vi "Dir Watch.vi"(8 "error in (no error)":errorcluster, 11 "System Data":T1={"System"={"Active"=FALSE, "Exit"=FALSE, "Command wait"="", "Status_Time"=0, "Time_GPS"=0}, "Stepper Motor"={"Connection Reference"="", "Valid Connection"=FALSE, "Speed"=15}, "Camera Data"={"Image path"=path "", "Filenames"=[], "Filenames queue"=[]}, "Core"={"Close Panel on Exit?"=FALSE, "Current VI Reference"=refnum}} {"Stepper Motor"."Speed" scale=0.0..30.0}) -> (0 "error out":errorcluster, 2 "Event Refnum":refnum<event-registration>, 3 "System Data out":T1={"System"={"Active"=FALSE, "Exit"=FALSE, "Command wait"="", "Status_Time"=0, "Time_GPS"=0}, "Stepper Motor"={"Connection Reference"="", "Valid Connection"=FALSE, "Speed"=15}, "Camera Data"={"Image path"=path "", "Filenames"=[], "Filenames queue"=[]}, "Core"={"Close Panel on Exit?"=FALSE, "Current VI Reference"=refnum}} {"Stepper Motor"."Speed" scale=0.0..30.0})   [LabVIEW 2019]
uses:
  System Data.ctl
  Stepper Data.ctl
  Camera Data.ctl
panel:
  out "user event out":refnum<user-event>
  in  "Files":i32(listbox) caption="Files (Only files are shown, not folders)"
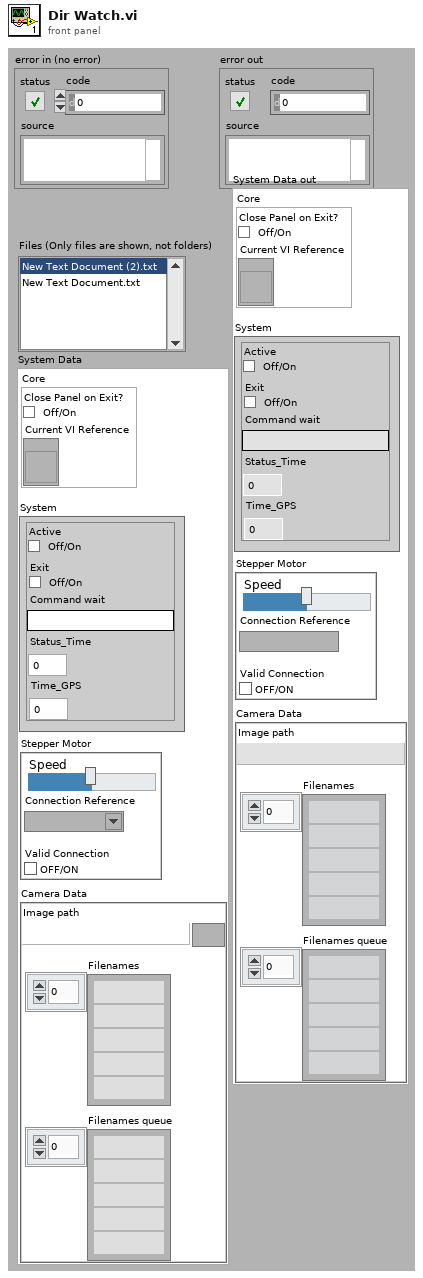
[diagram p1: front panel]
types:
  T1 = typedef "System Data.ctl" = cluster{"System":cluster{"Active":bool, "Exit":bool, "Command wait":string, "Status_Time":i32, "Time_GPS":i32}, "Stepper Motor":T2, "Camera Data":T3, "Core":cluster{"Close Panel on Exit?":bool, "Current VI Reference":refnum<vi>}}
  T2 = typedef "Stepper Data.ctl" = cluster{"Connection Reference":refnum<visa-resource-name>, "Valid Connection":bool, "Speed":i32}
  T3 = typedef "Camera Data.ctl" = cluster{"Image path":path, "Filenames":string[], "Filenames queue":string[]}
  T4 = cluster{"Dir Event":refnum<user-event>, "Image path":path}
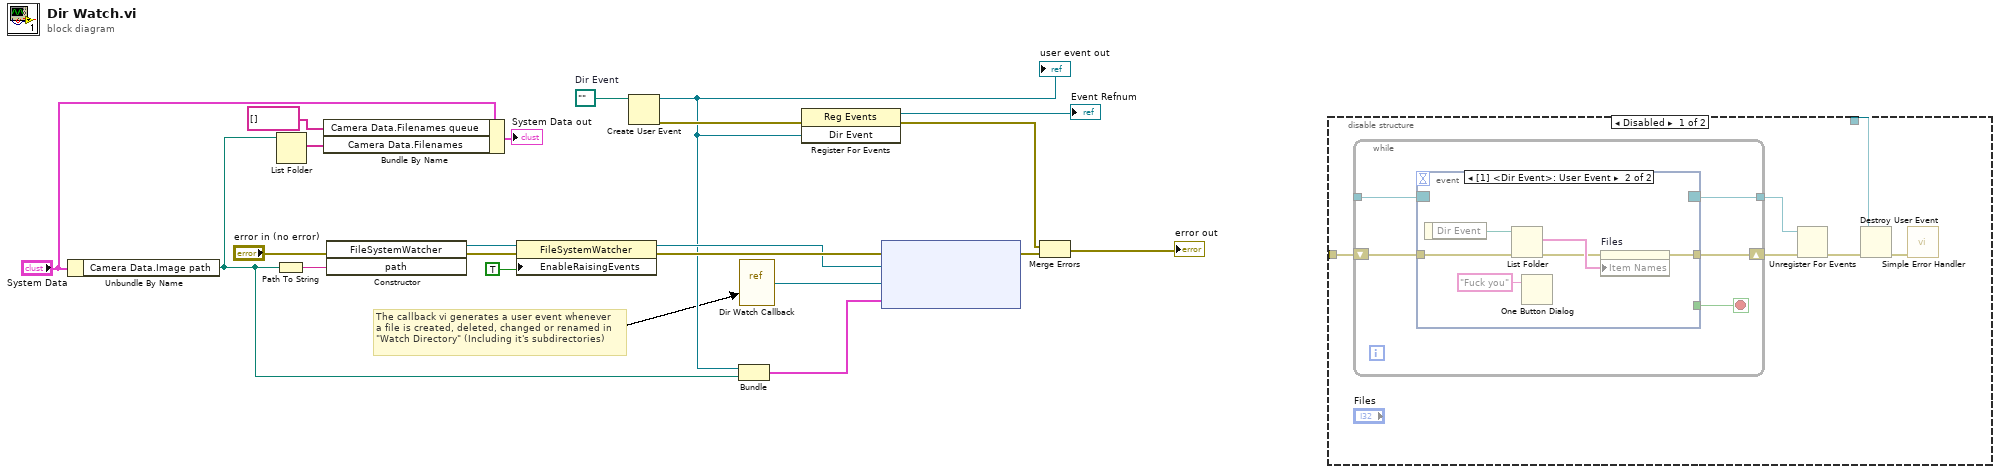
[diagram p0: block diagram]
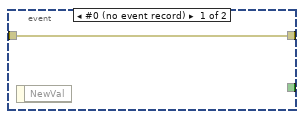
[diagram p2: hidden frame]
diagram:
  w9 = path ""  # Dir Event
  # "The callback vi generates a user event whenever\na file is created, deleted, changed or renamed in\n\"Watch Directory\" (Including it's subdirectories)"
  n1 = Unbundle By Name("System Data") -> ("Camera Data.Image path"=w5:path)
  n2 = Path To String(path=w5) -> (string=w17:string)
  n3 = List Folder(path=w5) -> (filenames=w3:string[])  [unwired: 3 in, 3 out]
  n4 = Bundle By Name(cluster="System Data", "Camera Data.Filenames queue"=string[] [], "Camera Data.Filenames"=w3) -> (→"System Data out":T1)
  n5 = constructor class="FileSystemWatcher"(error in="error in (no error)", "path"=w17) -> (reference out=w20:refnum<k24>, error out=w18:errorcluster)  [unwired: 2 in, 2 out]
  n6 = property class="FileSystemWatcher"(reference=w20, error in=w18, "EnableRaisingEvents"=TRUE) -> (reference out=w12:refnum<k24>, error out=w21:errorcluster)
  n7 = Create User Event(user event datatype=w9) -> (user event=w7:refnum<user-event>, error out=w16:errorcluster)  [unwired: 1 in]
  "user event out" <- w7
  n8 = Bundle("Dir Event"=w7, "Image path"=w5) -> (w11:T4)  [unwired: 1 in]
  n9 = vi-ref "Dir Watch Callback.vi"() -> ("vi reference"=w10:refnum<vi>)
  n10 = register-events(error in=w16, w7) -> (reference out=→"Event Refnum":refnum<event-registration>, error out=w14:errorcluster)  [unwired: 1 in]
  n11 = node(w21, w12, w10, w11) -> (w15:errorcluster)  [unwired: 1 in, 1 out]
  n12 = Merge Errors(w14, w15) -> (→"error out":errorcluster)
  n13 = disable-structure shown="Disabled" {
    disable-tunnel: _ -> [w23 _]
    disable-tunnel: _ -> [w22 _]
    frame Disabled {
      n14 = while {
        tunnel: _ -> [w31]
        shift-right: [w29] -> w26
        shift-left: w23 -> [w30]
        tunnel: [w28] -> w27
        stop <- w32 stop-if-true
        n15 = event shown="[1] <Dir Event>: User Event" {
          selector: w31 -> [_ _]
          dyn-events: [_ _] -> w28
          timeout: _ -> [_ _]
          tunnel: [w34 _] -> w32
          tunnel: w30 -> [w33 w40]
          tunnel: [w33 w36] -> w29
          event #0 (no event record) {
            n16 = event-data() -> ()  [unwired: 1 in, 1 out]
          }
          event User Event {
            n17 = event-data() -> ("Dir Event"=w39:path)  [unwired: 1 in]
            n18 = List Folder(path=w39, error in=w40) -> (filenames=w38:string[], error out=w37:errorcluster)  [unwired: 2 in, 2 out]
            n19 = One Button Dialog(message="Fuck you") -> ()  [unwired: 1 in, 1 out]
            n20 = property on="Files" class="LstBox (strict)"(error in=w37, "Item Names"=w38) -> (error out=w36:errorcluster)  [unwired: 1 in, 1 out]
          }
        }
      }
      n21 = Unregister For Events(event registration refnum=w27, error in=w26) -> (error out=w25:errorcluster)
      n22 = Destroy User Event(user event=w22, error in=w25) -> (error out=w24:errorcluster)
      n23 = call <vilib>:"Simple Error Handler.vi"("error in (no error)"=w24) -> ()  [unwired: 4 in, 5 out]
    }
    frame Enabled {
    }
  }
